vi "滚动字幕 (子VI).vi"(6 "停止按钮输入":bool, 9 "滚动方式":enum32{"左", "暂停", "右"}(radio), 10 "字幕内容":string="加油好男儿", 11 "滚动速度":u32=10) -> (2 "停止按钮输出":bool, 3 "?":bool[][](array[boolean]))   [LabVIEW 2018]
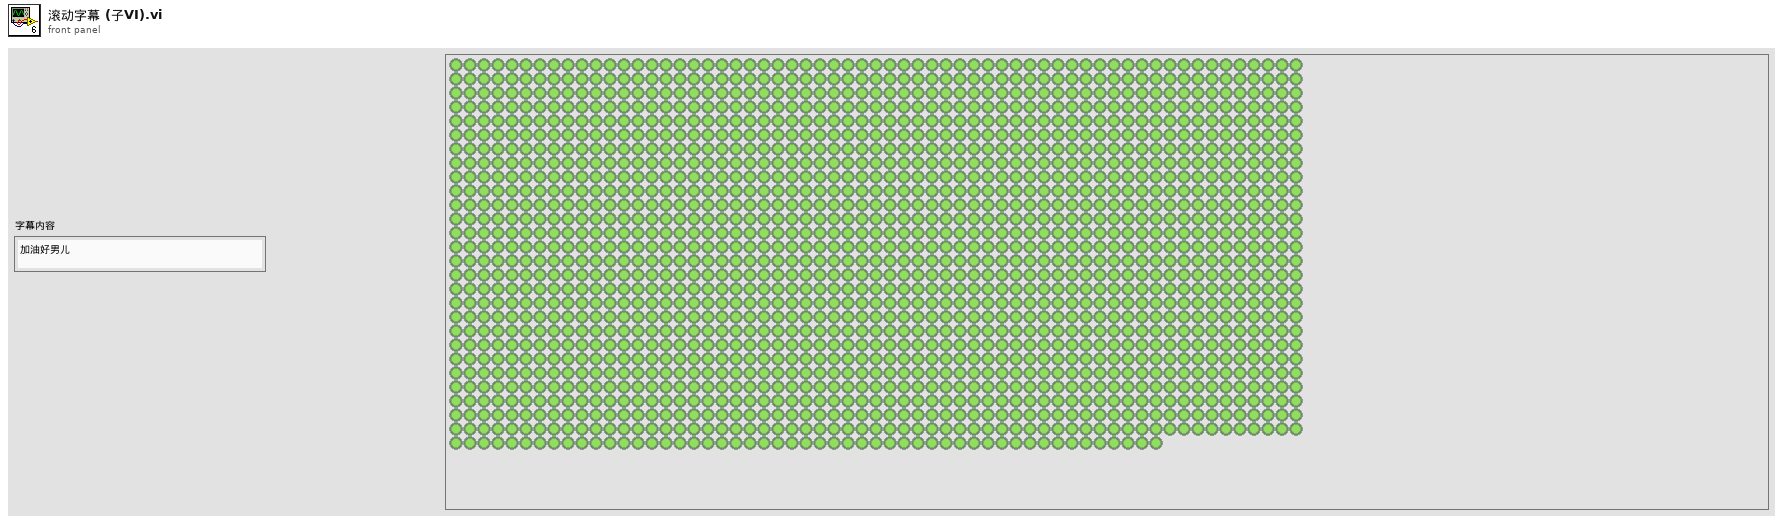
[diagram p1: front panel]
types:
  T1 = cluster{"left":i16, "top":i16, "right":i16, "bottom":i16}
  T2 = cluster{"Font Name:":string, "Size":i16, "Strikeout?":bool, "Italic?":bool, "Underline?":bool, "Outline?":bool, "Shadow?":bool, "Bold?":bool}
  T3 = enum16{"User-specified Font", "Application Font", "System Font", "Dialog Font"}
  T4 = typedef "imagedata.ctl" = cluster{"image type":i32, "image depth":i32, "image":u8[], "mask":u8[], "colors":u32[], "Rectangle":cluster{"left":i16, "top":i16, "right":i16, "bottom":i16}}
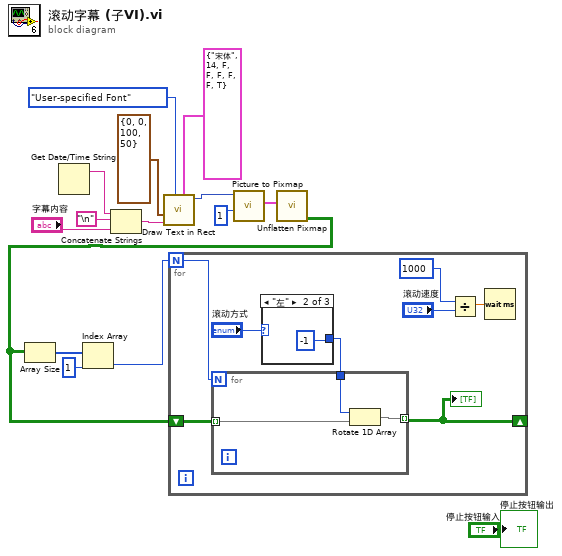
[diagram p0: block diagram]
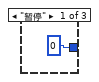
[diagram p2: hidden frame]
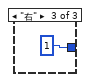
[diagram p3: hidden frame]
diagram:
  n1 = Get Date/Time String() -> (date string=w14:string)  [unwired: 3 in, 1 out]
  n2 = Concatenate Strings(w14, "\n", "字幕内容") -> (w4:string)
  n3 = call <vilib>:"Draw Text in Rect.vi"("[user-specified font]"=T2 {"Font Name:"="宋体", "Size"=14, "Strikeout?"=FALSE, "Italic?"=FALSE, "Underline?"=FALSE, "Outline?"=FALSE, "Shadow?"=FALSE, "Bold?"=TRUE}, "desired font(Application)"=T3."User-specified Font", "text"=w4, "rect"=T1 {"left"=0, "top"=0, "right"=100, "bottom"=50}) -> ("new picture"=w1:picture)  [unwired: 7 in]
  n4 = call <vilib>:"Picture to Pixmap.vi"("depth"=1, "picture"=w1) -> ("image data"=w2:T4)  [unwired: 8 in, 1 out]
  n5 = call <vilib>:"Unflatten Pixmap.vi"("image data"=w2) -> ("1-bit pixmap"=w9:bool[][])  [unwired: 4 in, 6 out]
  n6 = Array Size(array=w9) -> (size(s)=w6:i32[])
  n7 = Index Array(array=w6, index=1 ("索引")) -> (element=w8:i32)
  n8 = for {
    N: w8 -> [w22]
    shift-right: [w21] -> _
    shift-left: w9 -> [w23]
    n9 = case shown="\"左\"" "滚动方式" {
      tunnel: [0 -1 1] -> w16
      frame "暂停" {
      }
      frame "左" {
      }
      frame "右" {
      }
    }
    n10 = for {
      N: w22 -> [_]
      tunnel: w23 -> [w29] mode=indexing
      tunnel: [w28] -> w21 mode=indexing
      tunnel: w16 -> [w27]
      n11 = Rotate 1D Array(1:w29, 2:w27) -> (0:w28:bool[])
    }
    "?" <- w21
    n12 = Divide(x=u32 1000 ("y"), y="滚动速度") -> (x/y=w20:dbl)
    n13 = Wait (ms)(milliseconds to wait=w20) -> ()  [unwired: 1 out]
  }
  "停止按钮输出" <- "停止按钮输入"
